vi "tm3samp_03_acquirereplay.vi"() -> ()   [LabVIEW 2011]
panel:
  out "Image":u16[][](graph)
  in  "Play":bool
  in  "Acquire":bool
  out "Current Frame Index":i32=-1
  in  "Frames to Capture":i32=100
  out "Camera Serial":string
  out "Camera Model":string
  out "Camera Version":string
  out "Total Frames":i32
  out "error out":errorcluster {"code" format="%.0x"}
  in  "quit":bool
  # "This is an example of how to capture\ndata at full speed to RAM, then read \nthe data from the buffer later."
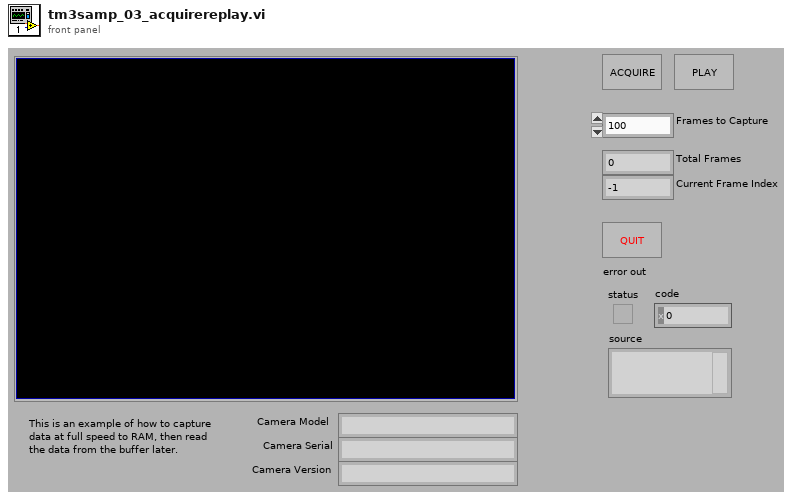
[diagram p1: front panel]
types:
  T1 = cluster{"Model":string, "Camera ID":string, "Firmware":string}
  T2 = cluster{"height":u32, "width":u32, "datatype":u32}
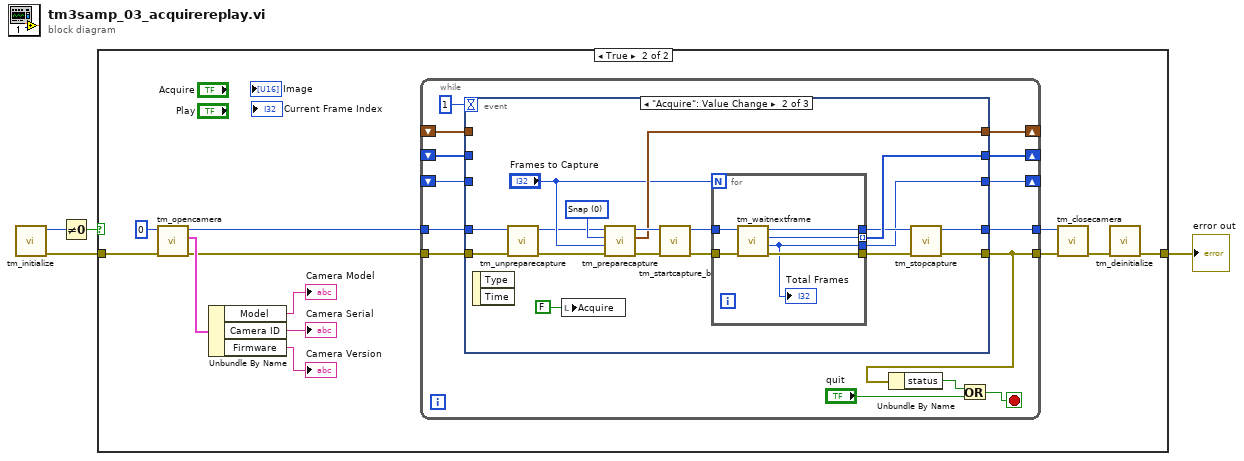
[diagram p0: block diagram]
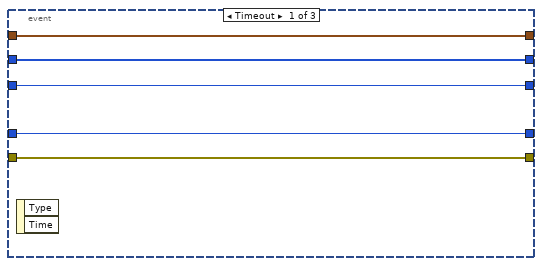
[diagram p3: hidden frame]
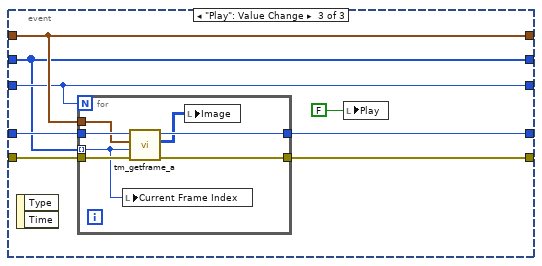
[diagram p4: hidden frame]
diagram:
  n1 = call <userlib>:"tm_initialize.vi"() -> ("error out"=w1:errorcluster, "Number Of Cameras"=w2:u32)  [unwired: 8 in, 2 out]
  n2 = Not Equal To 0?(x=w2) -> (x != 0?=w4:bool)
  n3 = case shown="True" w4 {
    tunnel: [w5 w14] -> w3
    tunnel: w1 -> [w5 w17]
    frame False {
    }
    frame True {
      n4 = call <userlib>:"tm_opencamera.vi"("error in (no error)"=w17, "Camera Index"=u32 0) -> ("error out"=w9:errorcluster, "Camera Details"=w10:T1, "Handle out"=w13:u32)  [unwired: 7 in]
      n5 = Unbundle By Name(w10) -> ("Model"=→"Camera Model":string, "Camera ID"=→"Camera Serial":string, "Firmware"=→"Camera Version":string)
      n6 = while {
        tunnel: [w22] -> w12
        tunnel: [w31] -> w11
        tunnel: w13 -> [w29]
        tunnel: w9 -> [w28]
        shift-right: [w18] -> _
        shift-left: _ -> [w25]
        shift-right: [w27] -> _
        shift-left: _ -> [w26]
        shift-right: [w24] -> _
        shift-left: _ -> [w23]
        stop <- w19 stop-if-true
        n7 = event shown="[1] \"Acquire\": Value Change" {
          selector: _ -> [_ _ _]
          dyn-events: _ -> [_ _ _]
          timeout: 1 -> [_ _ _]
          tunnel: [w35 w44 w68] -> w31
          tunnel: [w36 w45 w67] -> w22
          tunnel: w28 -> [w36 w40 w64]
          tunnel: w29 -> [w35 w37 w65]
          tunnel: [w34 w49 w66] -> w27
          tunnel: w26 -> [w34 _ w66]
          tunnel: [w32 w41 w63] -> w18
          tunnel: w25 -> [w32 _ w63]
          tunnel: [w33 w48 w61] -> w24
          tunnel: w23 -> [w33 _ w61]
          event Timeout {
            n8 = event-data() -> ()  [unwired: 1 in, 2 out]
          }
          event "Acquire": Value Change {
            w50 = 0 items=["Snap", "Sequence"] ("Capture mode")
            n9 = event-data() -> ()  [unwired: 1 in, 2 out]
            n10 = call <userlib>:"tm_unpreparecapture.vi"("error in (no error)"=w40, "Handle in"=w37) -> ("error out"=w39:errorcluster, "Handle out"=w38:u32)  [unwired: 8 in]
            n11 = local write "Acquire"(FALSE) -> ()
            n12 = call <userlib>:"tm_preparecapture.vi"("error in (no error)"=w39, "Frames"="Frames to Capture", "Capture mode"=w50, "Handle in"=w38) -> ("error out"=w51:errorcluster, "Buffer Info"=w49:T2, "Handle out"=w52:u32)  [unwired: 4 in, 1 out]
            n13 = call <userlib>:"tm_startcapture_b.vi"("error in (no error)"=w51, "Handle in"=w52) -> ("error out"=w53:errorcluster, "Handle out"=w54:u32)  [unwired: 8 in]
            n14 = for {
              N: "Frames to Capture" -> [_]
              tunnel: w53 -> [w59]
              tunnel: w54 -> [w60]
              tunnel: [w57] -> w48 mode=indexing
              tunnel: [w58] -> w43
              tunnel: [w55] -> w41
              tunnel: [w56] -> w42
              n15 = call <userlib>:"tm_waitnextframe.vi"("error in (no error)"=w59, "Handle in"=w60) -> ("error out"=w56:errorcluster, "Frame Count"=w55:i32, "Frame Index"=w57:i32, "Handle out"=w58:u32)  [unwired: 6 in]
              "Total Frames" <- w55
            }
            n16 = call <userlib>:"tm_stopcapture.vi"("error in (no error)"=w42, "Handle in"=w43) -> ("error out"=w45:errorcluster, "Handle out"=w44:u32)  [unwired: 8 in]
          }
          event "Play": Value Change {
            n17 = event-data() -> ()  [unwired: 1 in, 2 out]
            n18 = for {
              N: w63 -> [_]
              tunnel: w61 -> [w70] mode=indexing
              tunnel: w64 -> [w75]
              tunnel: w65 -> [w74]
              tunnel: w66 -> [w69]
              tunnel: [w73] -> w67
              tunnel: [w72] -> w68
              n19 = local write "Current Frame Index"(w70) -> ()
              n20 = call <userlib>:"tm_getframe_a.vi"("error in (no error)"=w75, "Frame Index"=w70, "Buffer Info"=w69, "Handle in"=w74) -> ("error out"=w73:errorcluster, "Data 16"=w71:u16[][], "Handle out"=w72:u32)  [unwired: 3 in, 2 out]
              n21 = local write "Image"(w71) -> ()
            }
            n22 = local write "Play"(FALSE) -> ()
          }
        }
        n23 = Unbundle By Name(w22) -> ("status"=w21:bool)
        n24 = Or(x=w21, y="quit") -> (x .or. y?=w19:bool)
      }
      n25 = call <userlib>:"tm_closecamera.vi"("error in (no error)"=w12, "Handle in"=w11) -> ("error out"=w15:errorcluster)  [unwired: 9 in]
      n26 = call <userlib>:"tm_deinitialize.vi"("error in (no error)"=w15) -> ("error out"=w14:errorcluster)  [unwired: 10 in]
    }
  }
  "error out" <- w3
